vi "jsonParseI64.vi"(8 "error in (no error)":errorcluster, 9 "default":i64, 10 "path":string, 11 "d in":i64) -> (0 "error out":errorcluster, 1 "found?":bool, 2 "value":i64, 3 "d out":i64)   [LabVIEW 2016, in "JSON Document.lvclass"]
uses:
  API/JSON Document Class/JSON Document.lvclass
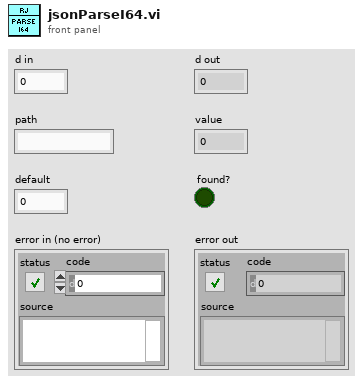
[diagram p1: front panel]
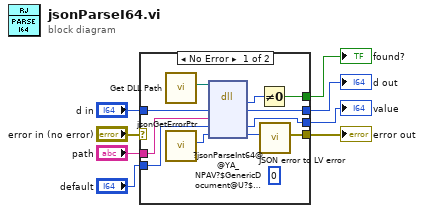
[diagram p0: block diagram]
diagram:
  n1 = case shown="No Error" "error in (no error)" {
    selector: "error in (no error)" -> [_ w22]
    tunnel: [w17 w22] -> w8
    tunnel: [w14 w21] -> w6
    tunnel: "default" -> [w15 w21]
    tunnel: [w13 w20] -> w4
    tunnel: "d in" -> [w12 w20]
    tunnel: "path" -> [w11 _]
    tunnel: [w10 _] -> w1
    frame No Error {
      (unwired) 0 ("found")
      n2 = call "Get DLL Path.vi"() -> ("Path"=w19:path)  [unwired: 11 in]
      n3 = call "jsonGetErrorPtr.vi"() -> ("return type"=w16:i64)  [unwired: 10 in, 1 out]
      n4 = dll-call lib="C:/Users/tblair/Documents/Git Projects/rapidjson-for-LabVIEW/lvrjs/Debug/lvrjs.dll" fn="?jsonParseInt64@@YA_NPAV?$GenericDocument@U?$UTF8@D@rapidjson@@V?$MemoryPoolAllocator@VCrtAllocator@rapidjson@@@2@VCrtAllocator@2@@rapidjson@@PADAA_J0@Z"(path in=w19, "d"=w12, "path"=w11, "value"=w15, "jsonError"=w16) -> ("return type"=w9:i32, "d"=w13:i64, "value"=w14:i64, "jsonError"=w18:i64)  [unwired: 3 in, 2 out]
      n5 = Not Equal To 0?(x=w9) -> (x != 0?=w10:bool)
      n6 = call "JSON error to LV error.vi"("jsonError"=w18) -> ("error out"=w17:errorcluster)  [unwired: 10 in]
    }
    frame Error {
    }
  }
  "error out" <- w8
  "value" <- w6
  "d out" <- w4
  "found?" <- w1
